vi "Read Module Index.vi"(8 "error in (no error)":errorcluster, 11 "RemIO Module in":refnum<class "RemIO Module.lvclass">) -> (0 "error out":errorcluster, 2 "Module Index":u8, 3 "RemIO Module out":refnum<class "RemIO Module.lvclass">)   [LabVIEW 2016, in "Modules.lvlib" / "RemIO Module.lvclass"]
uses:
  RemIO Module.lvclass
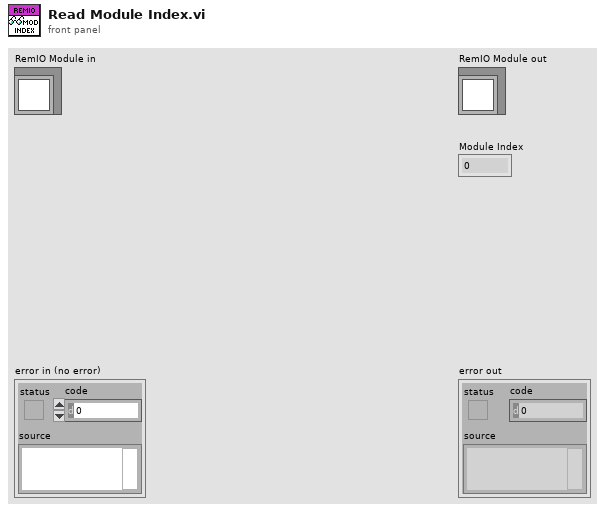
[diagram p1: front panel]
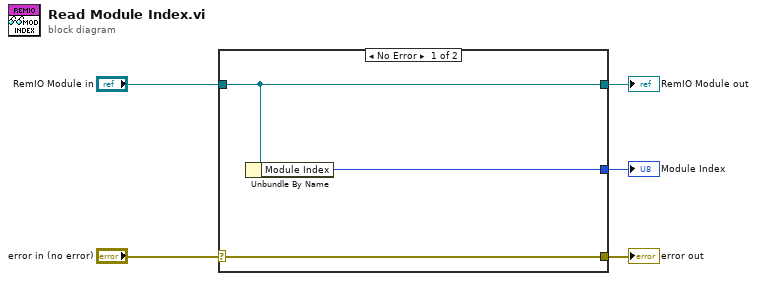
[diagram p0: block diagram]
diagram:
  n1 = case shown="No Error" "error in (no error)" {
    selector: "error in (no error)" -> [w8 w9]
    tunnel: [w8 w9] -> w4
    tunnel: [w7 w10] -> w2
    tunnel: "RemIO Module in" -> [w7 w10]
    tunnel: [w6 _] -> w1
    frame No Error {
      n2 = Unbundle By Name(w7) -> ("Module Index"=w6:u8)
    }
    frame Error {
    }
  }
  "error out" <- w4
  "RemIO Module out" <- w2
  "Module Index" <- w1
